vi "Prepare Acquisition.vi"(8 "error in (no error)":errorcluster, 10 "Camera Settings":T1={"Exposure Time (ms)"=100.0, "Binning"=enum."2x2", "Scan Mode"=0, "Frames to Acquire"=1000.0, "Pixel Correction"=FALSE, "Frames to Skip"=0, "File Path"=path "", "Duty cycle"=0.0, "ALEX"=FALSE, "Shutter Enable"=[], "fluidics trigger frame"=0, "Bit Depth"=0, "Image Width (px)"=0, "Image Height (px)"=0, "Horizontal Offset (px)"=0, "Vertical Offset (px)"=0} {"fluidics trigger frame" max=60000 step=1; "Exposure Time (ms)" min=1.0 max=10000.0 step=1.0}, 11 "Photometrics Camera in":refnum<class "Photometrics Camera.lvclass">) -> (0 "error out":errorcluster, 3 "Photometrics Camera out":refnum<class "Photometrics Camera.lvclass">)   [LabVIEW 2022 SP3, in "Photometrics Camera.lvlib" / "Photometrics Camera.lvclass"]
uses:
  Photometrics Camera.lvclass
  Resources/Type Defs/Camera Settings.ctl
  C:/FlashGordon/Development/dll/PVCamNET.dll
  dll/PVCamNET.dll
  Photometrics Camera.lvclass/Photometrics Camera.ctl
  Photometrics Camera.lvlib
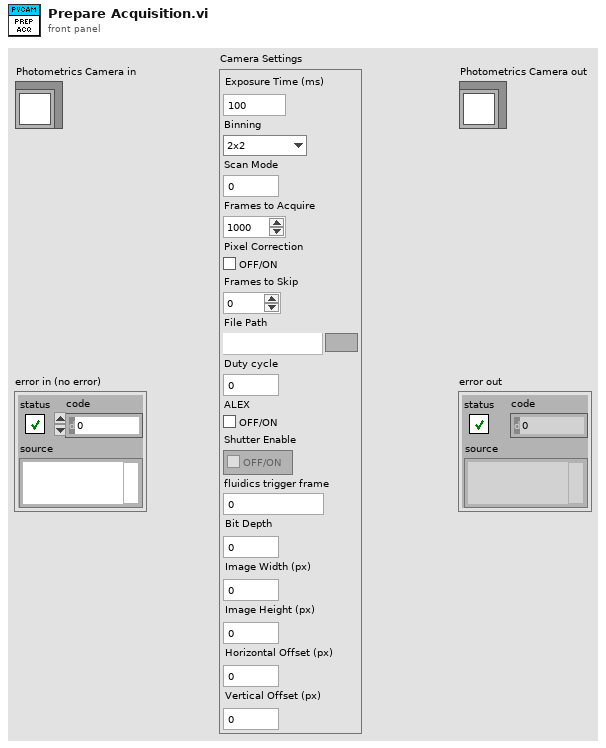
[diagram p1: front panel]
types:
  T1 = typedef "Camera Settings.ctl" = cluster{"Exposure Time (ms)":dbl, "Binning":enum16{"1x1", "2x2", "4x4"}, "Scan Mode":i32, "Frames to Acquire":dbl, "Pixel Correction":bool, "Frames to Skip":u32, "File Path":path, "Duty cycle":dbl, "ALEX":bool, "Shutter Enable":bool[], "fluidics trigger frame":u16, "Bit Depth":u16, "Image Width (px)":u16, "Image Height (px)":u16, "Horizontal Offset (px)":u16, "Vertical Offset (px)":u16}
  T2 = enum32{"Sensitivity (12-bit)", "Speed (8-bit)", "Dynamic Range (16-bit)", "Sub-Electron (16-bit)"}
  T3 = enum32{"First Row", "All Rows", "Any Row", "Rolling Shutter", "Line Output"}
  T4 = enum32{"Internal Trigger", "Edge Trigger", "Trigger First", "Level Trigger", "Level Trigger Overlap", "Software Trigger Edges", "Software Trigger First"}
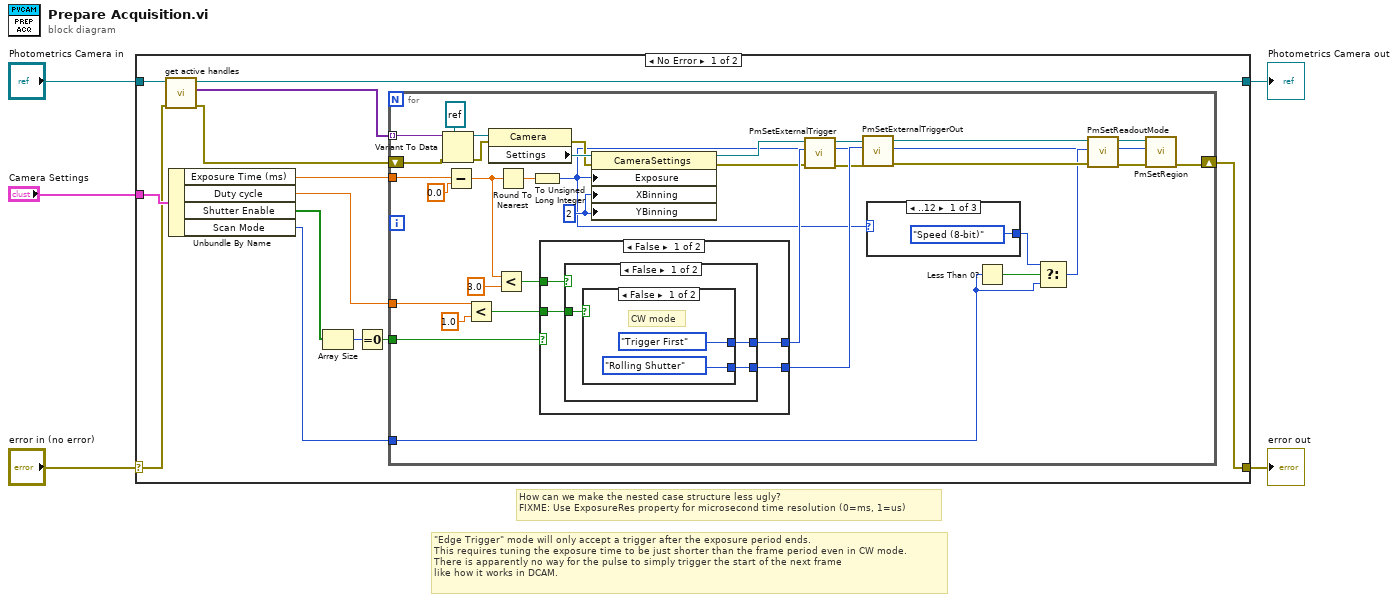
[diagram p0: block diagram]
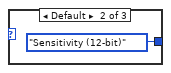
[diagram p2: hidden frame]
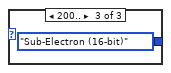
[diagram p3: hidden frame]
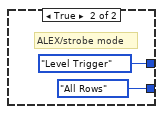
[diagram p4: hidden frame]
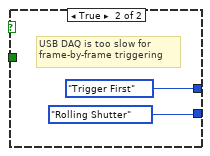
[diagram p5: hidden frame]
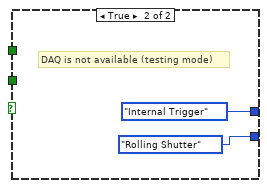
[diagram p6: hidden frame]
diagram:
  # "\"Edge Trigger\" mode will only accept a trigger after the exposure period ends.\nThis requires tuning the exposure time to be just shorter than the frame period even in CW mode.\nThere is apparently no way for the pulse to simply trigger the start of the next frame\nlike how it works in DCAM."
  # "How can we make the nested case structure less ugly?\nFIXME: Use ExposureRes property for microsecond time resolution (0=ms, 1=us)"
  n1 = case shown="No Error" "error in (no error)" {
    selector: "error in (no error)" -> [w8 w72]
    tunnel: [w18 w72] -> w4
    tunnel: [w10 w71] -> w2
    tunnel: "Photometrics Camera in" -> [w11 w71]
    tunnel: "Camera Settings" -> [w15 _]
    frame No Error {
      n2 = call-dynamic "get active handles.vi"("error in (no error)"=w8, "Camera in"=w11) -> ("error out"=w7:errorcluster, "Handles"=w9:variant[], "Camera out"=w10:refnum<class "Photometrics Camera.lvclass">)  [unwired: 5 in, 2 out]
      n3 = Unbundle By Name(w15) -> ("Exposure Time (ms)"=w17:dbl, "Duty cycle"=w16:dbl, "Shutter Enable"=w14:bool[], "Scan Mode"=w6:i32)
      n4 = Array Size(array=w14) -> (size(s)=w13:i32)
      n5 = Equal To 0?(x=w13) -> (x = 0?=w12:bool)
      n6 = for {
        shift-right: [w20] -> w18
        shift-left: w7 -> [w42]
        tunnel: w17 -> [w37]
        tunnel: w16 -> [w48]
        tunnel: w12 -> [w38]
        tunnel: w9 -> [w43] mode=indexing
        tunnel: w6 -> [w26]
        w50 = u16 2 ("XBinning")
        n7 = Variant To Data(error in=w42, type=refnum<k24> refnum ("reference out"), Variant=w43) -> (data=w40:refnum<k24>, error out=w41:errorcluster)
        n8 = Subtract(x=w37, y=0.0) -> (x-y=w36:dbl)
        n9 = Less?(x=w48, y=1.0) -> (x < y?=w46:bool)
        n10 = property class="Camera"(reference=w40, error in=w41) -> (error out=w51:errorcluster, "Settings"=w52:refnum<k24>)  [unwired: 1 out]
        n11 = Less?(x=w36, y=3.0) -> (x < y?=w44:bool)
        n12 = Round To Nearest(number=w36) -> (nearest integer value=w33:dbl)
        n13 = To Unsigned Long Integer(number=w33) -> (unsigned 32bit integer=w19:u32)
        n14 = case shown="False" w38 {
          tunnel: [w59 T4."Internal Trigger" ("Trigger Setting")] -> w49
          tunnel: w46 -> [w58 _]
          tunnel: w44 -> [w57 _]
          tunnel: [w56 T3."Rolling Shutter" ("Trigger Setting")] -> w34
          frame False {
            n15 = case shown="False" w57 {
              tunnel: [w62 T4."Trigger First" ("Trigger Setting")] -> w59
              tunnel: w58 -> [w61 _]
              tunnel: [w60 T3."Rolling Shutter" ("Trigger Setting")] -> w56
              frame False {
                n16 = case shown="False" w61 {
                  tunnel: [T4."Trigger First" ("Trigger Setting") T4."Level Trigger" ("Trigger Setting")] -> w62
                  tunnel: [T3."Rolling Shutter" ("Trigger Setting") T3."All Rows" ("Trigger Setting")] -> w60
                  frame False {
                    # "CW mode"
                  }
                  frame True {
                    # "ALEX/strobe mode"
                  }
                }
              }
              frame True {
                # "USB DAQ is too slow for \nframe-by-frame triggering"
              }
            }
          }
          frame True {
            # "DAQ is not available (testing mode)"
          }
        }
        n17 = property class="CameraSettings"(reference=w52, error in=w51, "Exposure"=w19, "XBinning"=w50, "YBinning"=w50) -> (reference out=w24:refnum<k24>, error out=w23:errorcluster)
        n18 = call "PmSetExternalTrigger.vi"("error in (no error)"=w23, "Trigger Setting"=w49, "reference"=w24) -> ("error out"=w31:errorcluster, "reference out"=w32:refnum<k24>)  [unwired: 7 in]
        n19 = call "PmSetExternalTriggerOut.vi"("error in (no error)"=w31, "Trigger Setting"=w34, "reference"=w32) -> ("error out"=w30:errorcluster, "reference out"=w29:refnum<k24>)  [unwired: 7 in]
        n20 = case shown="..12" w19 {
          tunnel: [T2."Speed (8-bit)" ("Trigger Setting") T2."Sensitivity (12-bit)" ("Trigger Setting") T2."Sub-Electron (16-bit)" ("Trigger Setting")] -> w27
          frame ..12 {
          }
          frame Default {
          }
          frame 200.. {
          }
        }
        n21 = Less Than 0?(x=w26) -> (x < 0?=w28:bool)
        n22 = Select(t=w27, s=w28, f=w26) -> (s? t:f=w25:u32)
        n23 = call "PmSetReadoutMode.vi"("error in (no error)"=w30, "Trigger Setting"=w25, "reference"=w29) -> ("error out"=w22:errorcluster, "reference out"=w21:refnum<k24>)  [unwired: 7 in]
        n24 = call "PmSetRegion.vi"("error in (no error)"=w22, "Exposure (ms)"=w19, "reference in"=w21) -> ("error out"=w20:errorcluster)  [unwired: 7 in, 1 out]
      }
    }
    frame Error {
    }
  }
  "error out" <- w4
  "Photometrics Camera out" <- w2
